vi "RSZVB Read Calibration Data.vi"(6 "Port 1 (1)":i32=1, 7 "Port 2 (1)":i32=1, 8 "error in (no error)":errorcluster {"code" format="%.0x"}, 9 "Error Term Parameters (0: Directivity)":i32(ring) items=["Directivity", "Source Match", "Reflection Tracking", "Reserved", "Load Match", "Transmission Tracking", "G11", "G12", "G21", "G22", "H11", "H12", "H21", "H22"], 10 "Channel (1)":i32=1, 11 "VISA session":refnum<visa-resource-name>) -> (0 "error out":errorcluster {"code" format="%.0x"}, 2 "Calibration Data":dbl[](array[numeric]) format="%^.3e", 3 "dup VISA session":refnum<visa-resource-name>)   [LabVIEW 2011]
doc: "This VI reads system error correction data for a specific channel, calibration method, and port combination <Port 1>, <Port 2>.\n\nRemote-control command(s):\nFORMat ASCII\nFORMat REAL,64\nSYSTem:COMMunicate:GPIB:SELF:RTERminator EOI\n[SENSe<Ch>:]CORRection:CDATa?"
uses:
  _utility/RSZVB Global Data.vi
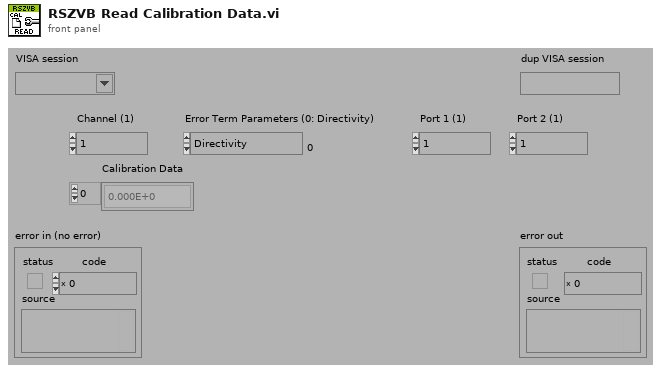
[diagram p1: front panel]
types:
  T1 = cluster{"Error Checking (T: On)":bool, "Installed Options":string[], "Data Valid?":bool, "Ports":i32, "Model":string[], "Option Checking (T: On)":bool}[]
  T2 = cluster{"Error Checking (T: On)":bool, "Installed Options":string[], "Data Valid?":bool, "Ports":i32, "Model":string[], "Option Checking (T: On)":bool}
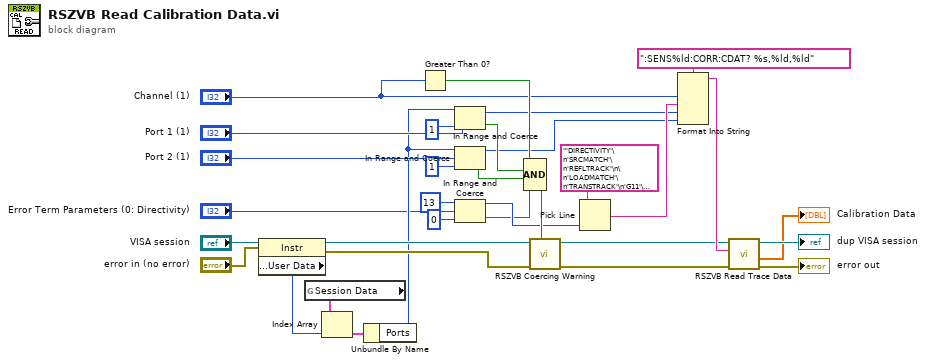
[diagram p0: block diagram]
diagram:
  n1 = property class="Instr"(reference="VISA session", error in="error in (no error)") -> (reference out=w26:refnum<visa-resource-name>, error out=w27:errorcluster, "General Settings:User Data"=w28:u32)
  n2 = global read "RSZVB Global Data.vi" "Session Data"() -> (w29:T1)
  n3 = Index Array(array=w29, index=w28) -> (element=w30:T2)
  n4 = Unbundle By Name(w30) -> ("Ports"=w11:i32)
  n5 = Greater Than 0?(x="Channel (1)") -> (x > 0?=w31:bool)
  n6 = In Range and Coerce(upper limit=w11, x="Port 1 (1)", lower limit=1) -> (coerced(x)=w8:i32, In Range?=w19:bool)
  n7 = In Range and Coerce(upper limit=w11, x="Port 2 (1)", lower limit=1) -> (coerced(x)=w7:i32, In Range?=w18:bool)
  n8 = In Range and Coerce(upper limit=13 ("lower limit"), x="Error Term Parameters (0: Directivity)", lower limit=0) -> (coerced(x)=w22:i32, In Range?=w17:bool)
  n9 = Compound Arithmetic op=AND(w31, w19, w18, w17) -> (w32:bool)
  n10 = call "RSZVB Coercing Warning.vi"("In Range?"=w32, "error in (no error)"=w27, "VISA session"=w26) -> ("error out"=w2:errorcluster, "dup VISA session"=w3:refnum<visa-resource-name>)  [unwired: 7 in]
  n11 = Pick Line(multi-line string="'DIRECTIVITY'\n'SRCMATCH'\n'REFLTRACK'\n\n'LOADMATCH'\n'TRANSTRACK'\n'G11'\n'G12'\n'G21'\n'G22'\n'H11'\n'H12'\n'H21'\n'H22'", line index=w22) -> (output string=w9:string)  [unwired: 1 in]
  n12 = Format Into String(format string=":SENS%ld:CORR:CDAT? %s,%ld,%ld", "Channel (1)", w9, w8, w7) -> (resulting string=w4:string)  [unwired: 2 in, 1 out]
  n13 = call "RSZVB Read Trace Data.vi"("error in (no error)"=w2, "Buffer"=w4, "VISA session"=w3) -> ("error out"=→"error out":errorcluster, "Trace Data"=→"Calibration Data":dbl[], "dup VISA session"=→"dup VISA session":refnum<visa-resource-name>)  [unwired: 6 in]
